vi "regexINI.vi"(8 "error in":errorcluster, 10 "INI String":string="[sectionName]\ntext = \"string\"\ncode = 123 // comment\n;code = 124\n\n[sectionName2]\ntext = \"string2\"\ncode = 345\n") -> (0 "error out":errorcluster, 2 "Sections":cluster{"section":string, "content":string}[](array[cluster]))   [LabVIEW 2013, in "CfgManager.Text.lvlib" / "ConfigManager.Text.INI.lvclass"]
uses:
  ConfigManager.Text.INI.lvclass
  <vilib>/regexp/Match Regular Expression.xnode
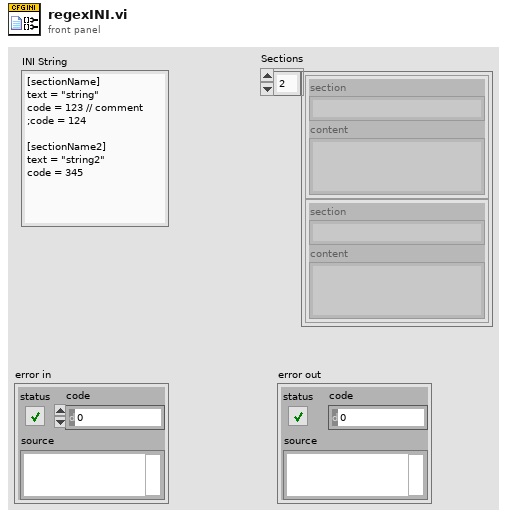
[diagram p1: front panel]
types:
  T1 = cluster{"submatch 1":string, "trimmed string":string}
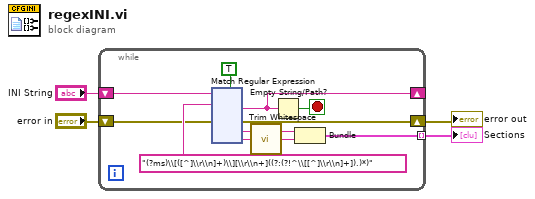
[diagram p0: block diagram]
diagram:
  n1 = while {
    shift-right: [w9] -> _
    shift-left: "INI String" -> [w15]
    tunnel: [w10] -> w3 mode=indexing
    shift-right: [w7] -> w1
    shift-left: "error in" -> [w6]
    stop <- w8 stop-if-true
    n2 = xnode "Match Regular Expression"("input string"=w15, "regular expression"="(?ms)\\[([^]\\r\\n]+)\\][\\r\\n+]((?:(?!^\\[[^]\\r\\n]+]).)*)" ("input string"), "error in"=w6, "multiline? (F)"=TRUE) -> ("after match"=w9:string, "error out"=w7:errorcluster, "submatch 1"=w13:string, "submatch 2"=w12:string)  [unwired: 2 in, 3 out]
    n3 = call <vilib>:"Trim Whitespace.vi"("string"=w12) -> ("trimmed string"=w11:string)  [unwired: 1 in]
    n4 = Empty String/Path?(string/path=w9) -> (empty?=w8:bool)
    n5 = Bundle("submatch 1"=w13, "trimmed string"=w11) -> (w10:T1)  [unwired: 1 in]
  }
  "Sections" <- w3
  "error out" <- w1
